vi "PlacePiece.vi"(1 "place":i32, 2 "player":i32, 3 "Board":i32[][](array[numeric])) -> (0 "board_out":i32[][](array[numeric]))   [LabVIEW 2025]
panel:
  out "row":i32
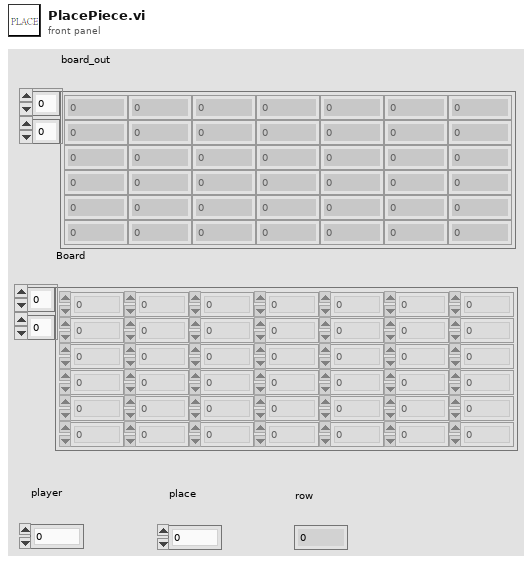
[diagram p1: front panel]
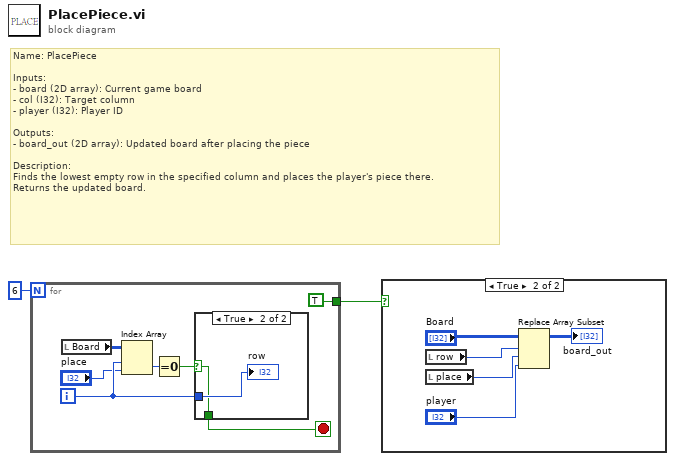
[diagram p0: block diagram]
diagram:
  # "Name: PlacePiece\n\nInputs:\n- board (2D array): Current game board\n- col (I32): Target column\n- player (I32): Player ID\n\nOutputs:\n- board_out (2D array): Updated board after placing the piece\n\nDescription:\nFinds the lowest empty row in the specified column and places the player's piece there.\nReturns the updated board."
  n1 = for {
    N: 6 -> [_]
    tunnel: [TRUE] -> w1
    i -> [w5]
    stop <- w7 stop-if-true
    n2 = local read "Board"() -> (w3:i32[][])
    n3 = Index Array(array=w3, index (row)=w5, index (col)="place") -> (element=w8:i32)
    n4 = Equal To 0?(x=w8) -> (x = 0?=w9:bool)
    n5 = case shown="True" w9 {
      selector: w9 -> [w10 w11]
      tunnel: w5 -> [_ w12]
      tunnel: [w10 w11] -> w7
      frame False {
      }
      frame True {
        "row" <- w12
      }
    }
  }
  n6 = case shown="True" w1 {
    frame False {
    }
    frame True {
      n7 = local read "row"() -> (w16:i32)
      n8 = local read "place"() -> (w15:i32)
      n9 = Replace Array Subset(array="Board", new element="player", index (row)=w16, index (col)=w15) -> (→"board_out":i32[][])
    }
  }
